vi "5.4_ClusterScaling.vi"() -> ()   [LabVIEW 2025]
panel:
  in  "Raw Data":T1
  out "Scaled Data":T2 {"Thermometer" scale=0.0..100.0; "pressure (N/m^2)" scale=0.0..10.0; "flow rate (liters/sec)" scale=0.0..10.0}
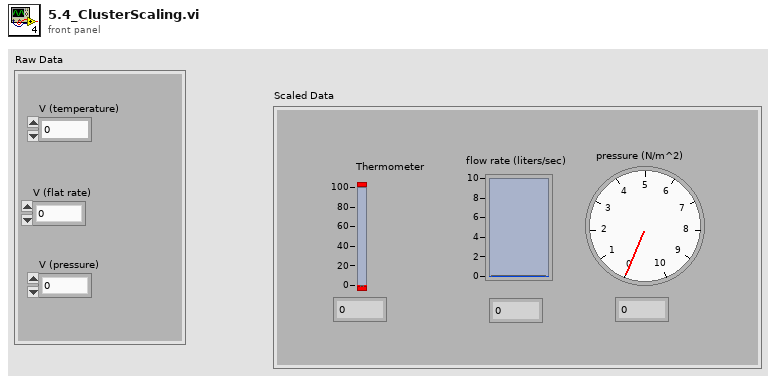
[diagram p1: front panel]
types:
  T1 = cluster{"V (temperature)":dbl, "V (flat rate)":dbl, "V (pressure)":dbl}
  T2 = cluster{"flow rate (liters/sec)":dbl, "pressure (N/m^2)":dbl, "Thermometer":dbl}
  T3 = cluster{"deg C/V":dbl, " (N/m^2)/ V":dbl, "(liters/sec)/V":dbl}
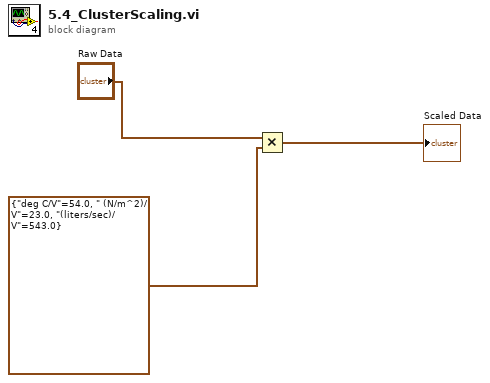
[diagram p0: block diagram]
diagram:
  n1 = Multiply(x="Raw Data", y=T3 {"deg C/V"=54.0, " (N/m^2)/ V"=23.0, "(liters/sec)/V"=543.0}) -> (x*y=→"Scaled Data":cluster{dbl, dbl, dbl})
